vi "VariantDemo.vi"() -> ()   [LabVIEW 2014]
panel:
  out "Cluster out":cluster{"Member 1":dbl, "Member 2":string}={"Member 1"=38.0, "Member 2"="foo bar"}
  out "Boolean Out":bool
  out "String Out":string
  out "I32 Out":i32
  out "Variant":variant
  in  "Selector":enum16{"I32", "String", "Boolean", "Cluster"}(ring)
  in  "Cluster":cluster{"Member 1":dbl, "Member 2":string}={"Member 1"=38.0, "Member 2"="foo bar"}
  in  "Boolean":bool
  in  "String":string="Hello, world!"
  in  "I32":i32=42
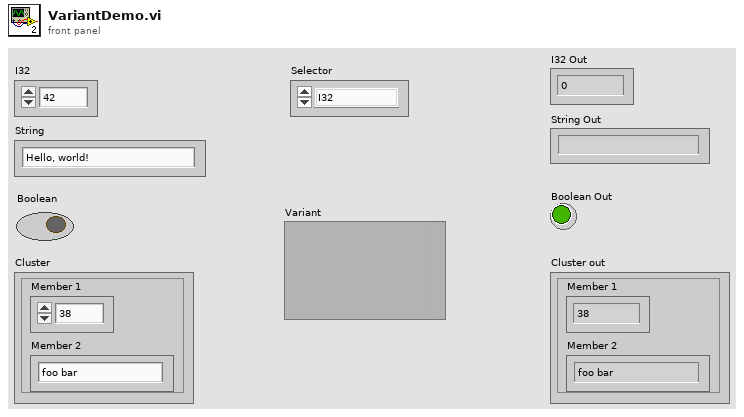
[diagram p1: front panel]
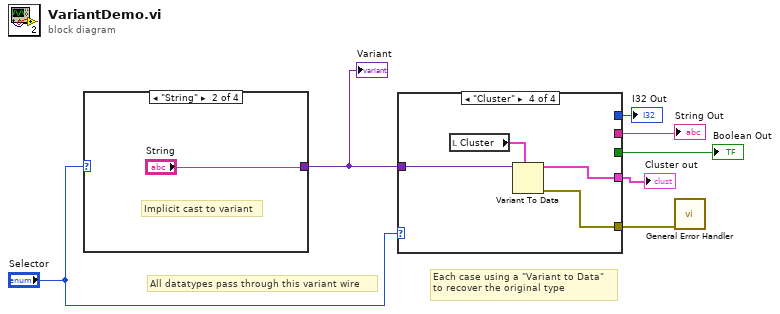
[diagram p0: block diagram]
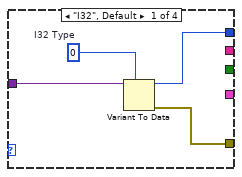
[diagram p2: hidden frame]
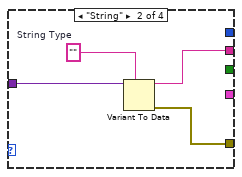
[diagram p3: hidden frame]
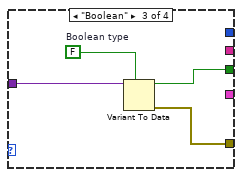
[diagram p4: hidden frame]
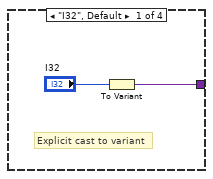
[diagram p5: hidden frame]
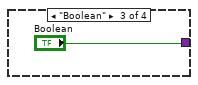
[diagram p6: hidden frame]
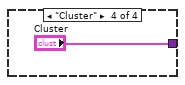
[diagram p7: hidden frame]
diagram:
  # "Each case using a \"Variant to Data\"\nto recover the original type"
  # "All datatypes pass through this variant wire"
  n1 = case shown="\"String\"" "Selector" {
    tunnel: [w8 "String" "Boolean" "Cluster"] -> w6
    frame "I32", Default {
      # "Explicit cast to variant"
      n2 = To Variant(anything="I32") -> (Variant=w8:variant)
    }
    frame "String" {
      # "Implicit cast to variant"
    }
    frame "Boolean" {
    }
    frame "Cluster" {
    }
  }
  "Variant" <- w6
  n3 = case shown="\"Cluster\"" "Selector" {
    tunnel: w6 -> [w16 w20 w24 w28]
    tunnel: [w14 _ _ _] -> w5
    tunnel: [w13 w18 w22 w27] -> w4
    tunnel: [_ w17 _ _] -> w3
    tunnel: [_ _ _ w25] -> w1
    tunnel: [_ _ w21 _] -> w2
    frame "I32", Default {
      w15 = 0  # I32 Type
      n4 = Variant To Data(type=w15, Variant=w16) -> (data=w14:i32, error out=w13:errorcluster)  [unwired: 1 in]
    }
    frame "String" {
      w19 = ""  # String Type
      n5 = Variant To Data(type=w19, Variant=w20) -> (data=w17:string, error out=w18:errorcluster)  [unwired: 1 in]
    }
    frame "Boolean" {
      w23 = FALSE  # Boolean type
      n6 = Variant To Data(type=w23, Variant=w24) -> (data=w21:bool, error out=w22:errorcluster)  [unwired: 1 in]
    }
    frame "Cluster" {
      n7 = local read "Cluster"() -> (w26:cluster{"Member 1":dbl, "Member 2":string})
      n8 = Variant To Data(type=w26, Variant=w28) -> (data=w25:cluster{"Member 1":dbl, "Member 2":string}, error out=w27:errorcluster)  [unwired: 1 in]
    }
  }
  "I32 Out" <- w5
  "String Out" <- w3
  "Boolean Out" <- w2
  "Cluster out" <- w1
  n9 = call <vilib>:"General Error Handler.vi"("error in (no error)"=w4) -> ()  [unwired: 10 in, 5 out]
